vi "MessageGenerator.vi"() -> ()   [LabVIEW 2017, in "MessageGen.lvlib"]
uses:
  <vilib>/addons/InsightCM/MessageBus/CodeGen/MessageGen.lvlib
  <vilib>/addons/InsightCM/MessageBus/CodeGen/controls/MessageData.ctl
  <vilib>/addons/InsightCM/MessageBus/CodeGen/controls/MessageType.ctl
  <vilib>/addons/InsightCM/MessageBus/CodeGen/controls/Parameter.ctl
  <vilib>/addons/InsightCM/MessageBus/CodeGen/controls/ParameterType.ctl
panel:
  out "Error Msgs":string[](array[string])
  out "Missing Ctls":string[](array[string])
  out "Messages":i32
  out "Iteration":i32
  out "Current Message":T1
  out "error out":errorcluster
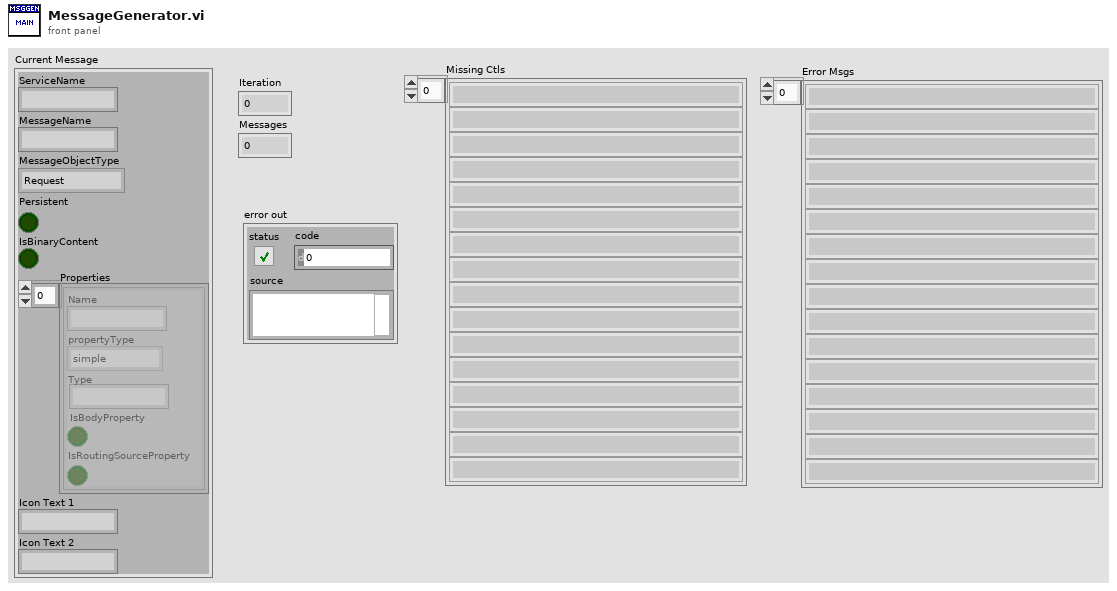
[diagram p1: front panel]
types:
  T1 = typedef "MessageGen.lvlib/MessageData.ctl" = cluster{"ServiceName":string, "MessageName":string, "MessageObjectType":T2, "Persistent":bool, "IsBinaryContent":bool, "Properties":T3[], "Icon Text 1":string, "Icon Text 2":string}
  T2 = typedef "MessageGen.lvlib/MessageType.ctl" = enum16{"Request", "Response", "Broadcast", "RoutedMessage"}
  T3 = typedef "MessageGen.lvlib/Parameter.ctl" = cluster{"Name":string, "propertyType":T4, "Type":string, "IsBodyProperty":bool, "IsRoutingSourceProperty":bool}
  T4 = typedef "MessageGen.lvlib/ParameterType.ctl" = enum16{"simple", "bytearray", "dateTime", "list", "map", "object"}
  T5 = typedef "MessageGen.lvlib/ServiceDef.ctl" = cluster{"Name":string, "Prefix":string, "MessageDefs":T6[]}
  T6 = typedef "MessageGen.lvlib/MessageDef.ctl" = cluster{"Name":string, "Type":string, "IconText1":string, "IconText2":string, "Persistent":bool, "ContentType":string, "Parameters":T7[], "ResultContentType":string, "Results":T7[]}
  T7 = typedef "MessageGen.lvlib/ParameterDef.ctl" = cluster{"Name":string, "Type":string, "ElementType":string}
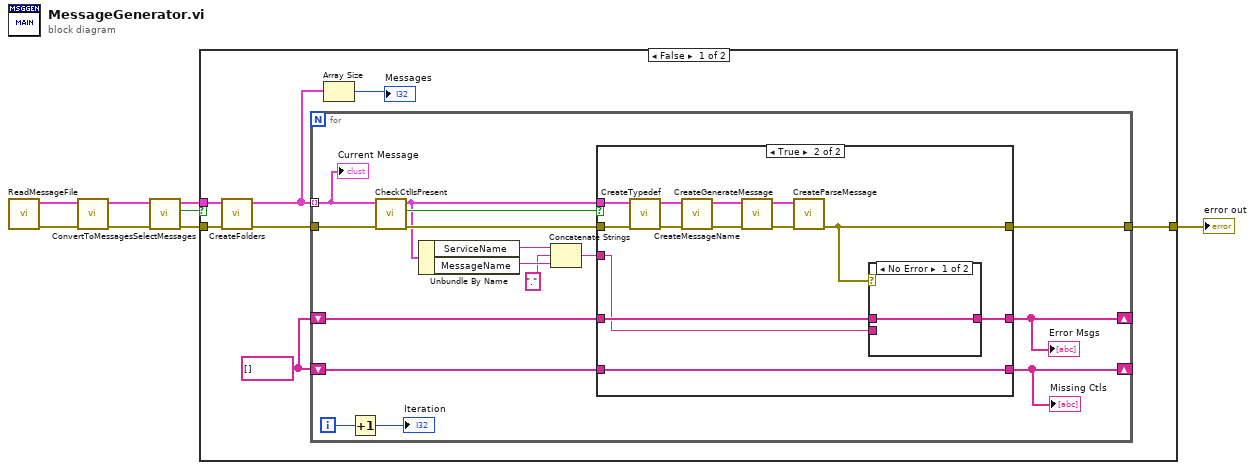
[diagram p0: block diagram]
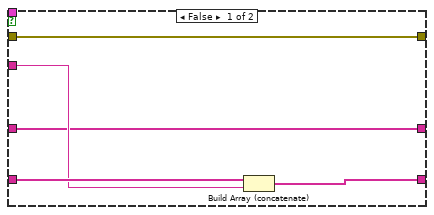
[diagram p2: hidden frame]
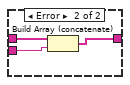
[diagram p3: hidden frame]
diagram:
  n1 = call <vilib>:"ReadMessageFile.vi"() -> ("error out"=w6:errorcluster, "ServiceDefs"=w8:T5[])  [unwired: 10 in]
  n2 = call <vilib>:"ConvertToMessages.vi"("error in (no error)"=w6, "ServiceDefs"=w8) -> ("error out"=w5:errorcluster, "Messages"=w7:T1[])  [unwired: 8 in]
  n3 = call <vilib>:"SelectMessages.vi"("error in (no error)"=w5, "Messages in"=w7) -> ("error out"=w4:errorcluster, "Cancelled"=w2:bool, "Messages out"=w3:T1[])  [unwired: 7 in]
  n4 = case shown="False" w2 {
    tunnel: w4 -> [w15 w54]
    tunnel: w3 -> [w14 _]
    tunnel: [w12 w54] -> w1
    frame False {
      w9 = string[] []
      n5 = call <vilib>:"CreateFolders.vi"("error in (no error)"=w15, "Messages in"=w14) -> ("error out"=w13:errorcluster, "Messages out"=w11:T1[])  [unwired: 8 in]
      n6 = for {
        tunnel: w11 -> [w27] mode=indexing
        shift-right: [w23] -> _
        shift-left: w9 -> [w24]
        tunnel: w13 -> [w28]
        tunnel: [w31] -> w12
        shift-right: [w16] -> _
        shift-left: w9 -> [w17]
        i -> [w30]
        n7 = Increment(x=w30) -> (x+1=→"Iteration":i32)
        n8 = call <vilib>:"CheckCtlIsPresent.vi"("error in (no error)"=w28, "Message"=w27) -> ("error out"=w26:errorcluster, "ctl present"=w25:bool, "Message"=w19:T1)  [unwired: 7 in]
        n9 = Unbundle By Name(w19) -> ("ServiceName"=w22:string, "MessageName"=w21:string)
        n10 = Concatenate Strings(w22, "." ("string"), w21) -> (w18:string)
        n11 = case shown="True" w25 {
          tunnel: [w36 w40] -> w31
          tunnel: w19 -> [_ w43]
          tunnel: w26 -> [w36 w42]
          tunnel: w24 -> [w35 w41]
          tunnel: [w34 w41] -> w23
          tunnel: w18 -> [w33 w37]
          tunnel: w17 -> [w32 w39]
          tunnel: [w32 w38] -> w16
          frame False {
            n12 = Build Array (concatenate)(w35, w33) -> (w34:string[])
          }
          frame True {
            n13 = call <vilib>:"CreateTypedef.vi"("error in (no error)"=w42, "Message in"=w43) -> ("error out"=w45:errorcluster, "Message out"=w47:T1)  [unwired: 8 in]
            n14 = call <vilib>:"CreateMessageName.vi"("error in (no error)"=w45, "Message in"=w47) -> ("error out"=w44:errorcluster, "Message out"=w46:T1)  [unwired: 8 in]
            n15 = call <vilib>:"CreateGenerateMessage.vi"("error in (no error)"=w44, "Message in"=w46) -> ("error out"=w49:errorcluster, "Message out"=w48:T1)  [unwired: 8 in]
            n16 = call <vilib>:"CreateParseMessage.vi"("error in (no error)"=w49, "Message in"=w48) -> ("error out"=w40:errorcluster)  [unwired: 8 in, 1 out]
            n17 = case shown="No Error" w40 {
              tunnel: w39 -> [w50 w53]
              tunnel: [w50 w52] -> w38
              tunnel: w37 -> [_ w51]
              frame No Error {
              }
              frame Error {
                n18 = Build Array (concatenate)(w53, w51) -> (w52:string[])
              }
            }
          }
        }
        "Missing Ctls" <- w23
        "Error Msgs" <- w16
        "Current Message" <- w27
      }
      n19 = Array Size(array=w11) -> (size(s)=→"Messages":i32)
    }
    frame True {
    }
  }
  "error out" <- w1
